vi "Resolve Template Variable.vi"(8 "error in (no error)":errorcluster, 10 "Variable Name":string, 11 "VolatusVariableResolver in":refnum<class "VolatusVariableResolver.lvclass">) -> (0 "error out":errorcluster, 2 "Value":string)   [LabVIEW 2020, in "Volatus.lvlib" / "VolatusVariableResolver.lvclass"]
uses:
  VolatusVariableResolver.lvclass
  VolatusVariableResolver.lvclass/VolatusVariableResolver.ctl
  VolatusAPI/VolatusAPI.lvclass
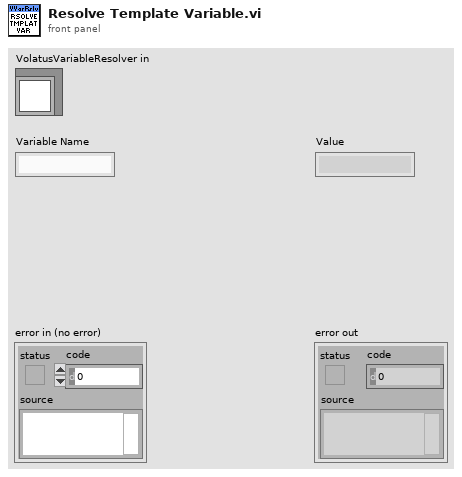
[diagram p1: front panel]
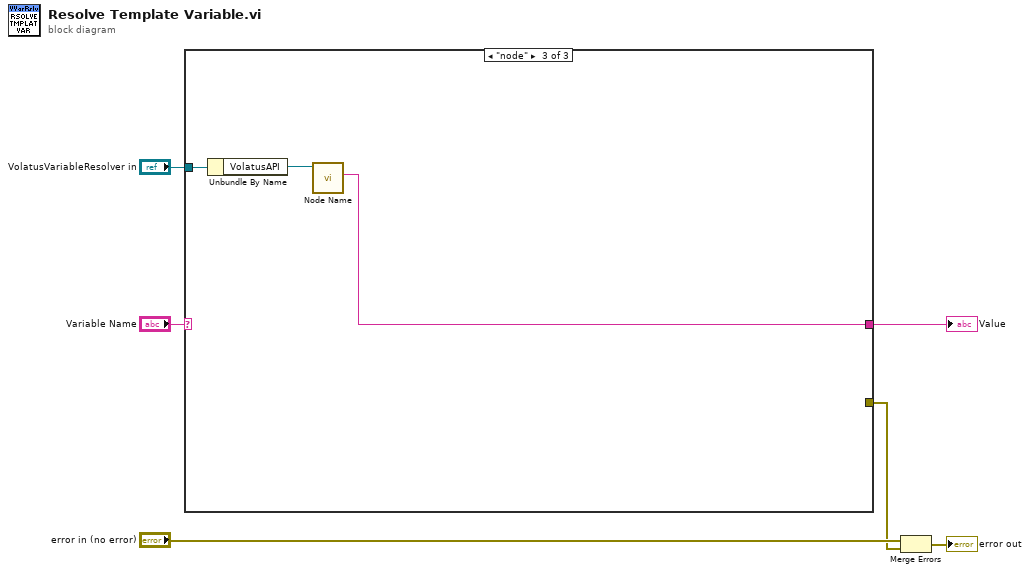
[diagram p0: block diagram]
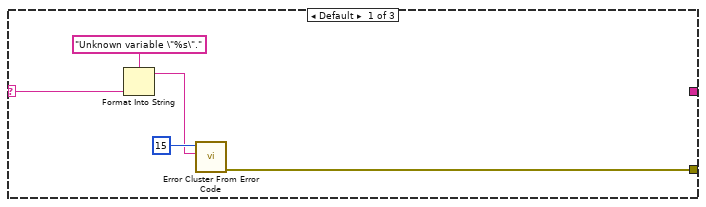
[diagram p2: hidden frame]
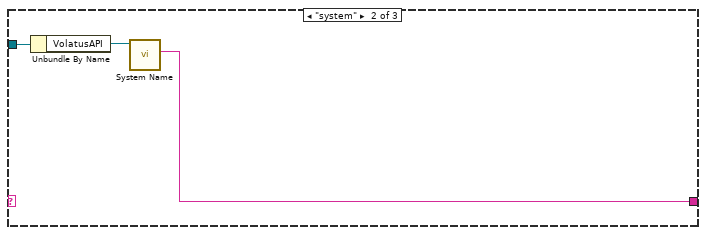
[diagram p3: hidden frame]
diagram:
  n1 = case shown="\"node\"" "Variable Name" {
    selector: "Variable Name" -> [w10 _ _]
    tunnel: "VolatusVariableResolver in" -> [_ w14 w17]
    tunnel: [_ w12 w15] -> w3
    tunnel: [w7 _ _] -> w1
    frame Default {
      n2 = Format Into String(format string="Unknown variable \"%s\".", w10) -> (resulting string=w8:string)  [unwired: 2 in, 1 out]
      n3 = call <vilib>:"Error Cluster From Error Code.vi"("error message (\"\")"=w8, "error code (0)"=15) -> ("error out"=w7:errorcluster)  [unwired: 7 in]
    }
    frame "system" {
      n4 = Unbundle By Name(w14) -> ("VolatusAPI"=w13:refnum<class "VolatusAPI.lvclass">)
      n5 = call "System Name.vi"("VolatusAPI in"=w13) -> ("System"=w12:string)  [unwired: 9 in, 1 out]
    }
    frame "node" {
      n6 = Unbundle By Name(w17) -> ("VolatusAPI"=w16:refnum<class "VolatusAPI.lvclass">)
      n7 = call "Node Name.vi"("VolatusAPI in"=w16) -> ("Node Name"=w15:string)  [unwired: 8 in, 2 out]
    }
  }
  "Value" <- w3
  n8 = Merge Errors("error in (no error)", w1) -> (→"error out":errorcluster)
